vi "5 ch 1 sample minimum resonance scanner (FPGA) fixed pix clock.vi"() -> ()   [LabVIEW 2012]
uses:
  <vilib>/eio/EIONode/EIONode.xnode
  <vilib>/rvi/eio/common/nirviEmuTemplateMethod_errors.vi
  <vilib>/rvi/DataTransferAndStorage/Container/XNode/niFpgaContainer.xnode
  <vilib>/platform/TimedLoop/XDataNode/XDataNode.xnode
  <vilib>/Platform/TimedLoop/XDataNode/nitl_modes.ctl
  <vilib>/Platform/TimedLoop/XDataNode/XDNodeRunTimeDep.lvlib
  <vilib>/Platform/TimedLoop/XDataNode/wakeup.ctl
  <vilib>/Platform/TimedLoop/XDataNode/timing_clust.ctl
  <vilib>/rvi/interface/RandomDataEmulation/nirviRandomDataFpgaReadWriteTemplate.vi
panel:
  in  "lines at once":i16=4999
  in  "samples per half period":i16=4999
  in  "Start Delay (Ticks)":i16 caption="Start delay (Ticks)"
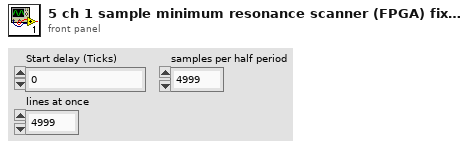
[diagram p1: front panel]
types:
  T1 = typedef "XDNodeRunTimeDep.lvlib/timing_clust.ctl" = cluster{"Expected End [f-1]":u64, "Actual End [f-1]":u64, "Finished Late? [f-1]":bool, "Expected End [i-1]":u64, "Actual End [i-1]":u64, "Finished Late? [i-1]":bool, "Expected Start [i]":u64, "Actual Start [i]":u64, "Expected Start [f]":u64, "Actual Start [f]":u64, "Source Name":string, "Structure Name":string, "Period":i64, "Deadline":i64, "Offset":i64, "Start":i64, "Priority":i32, "Timeout":i32, "Mode":T2, "Wakeup Reason":T3, "Error":errorcluster, "Source Type":string, "Secondary Source Type":string, "Global End Time":u64, "Global Start Time":u64, "Frame Duration":u64, "Iteration Duration":u64, "Assigned CPU":i32, "I/O Scan Engine Mode":u32}
  T2 = typedef "XDNodeRunTimeDep.lvlib/nitl_modes.ctl" = enum32{"No Change", "Process missed periods, maintain original phase", "Discard missed periods, maintain original phase", "Process missed periods, ignore original phase", "Discard missed periods, ignore original phase"}
  T3 = typedef "XDNodeRunTimeDep.lvlib/wakeup.ctl" = enum32{"Normal", "Aborted", "Asynchronous wakeup", "Timing source error", "Timed loop error", "Timeout"}
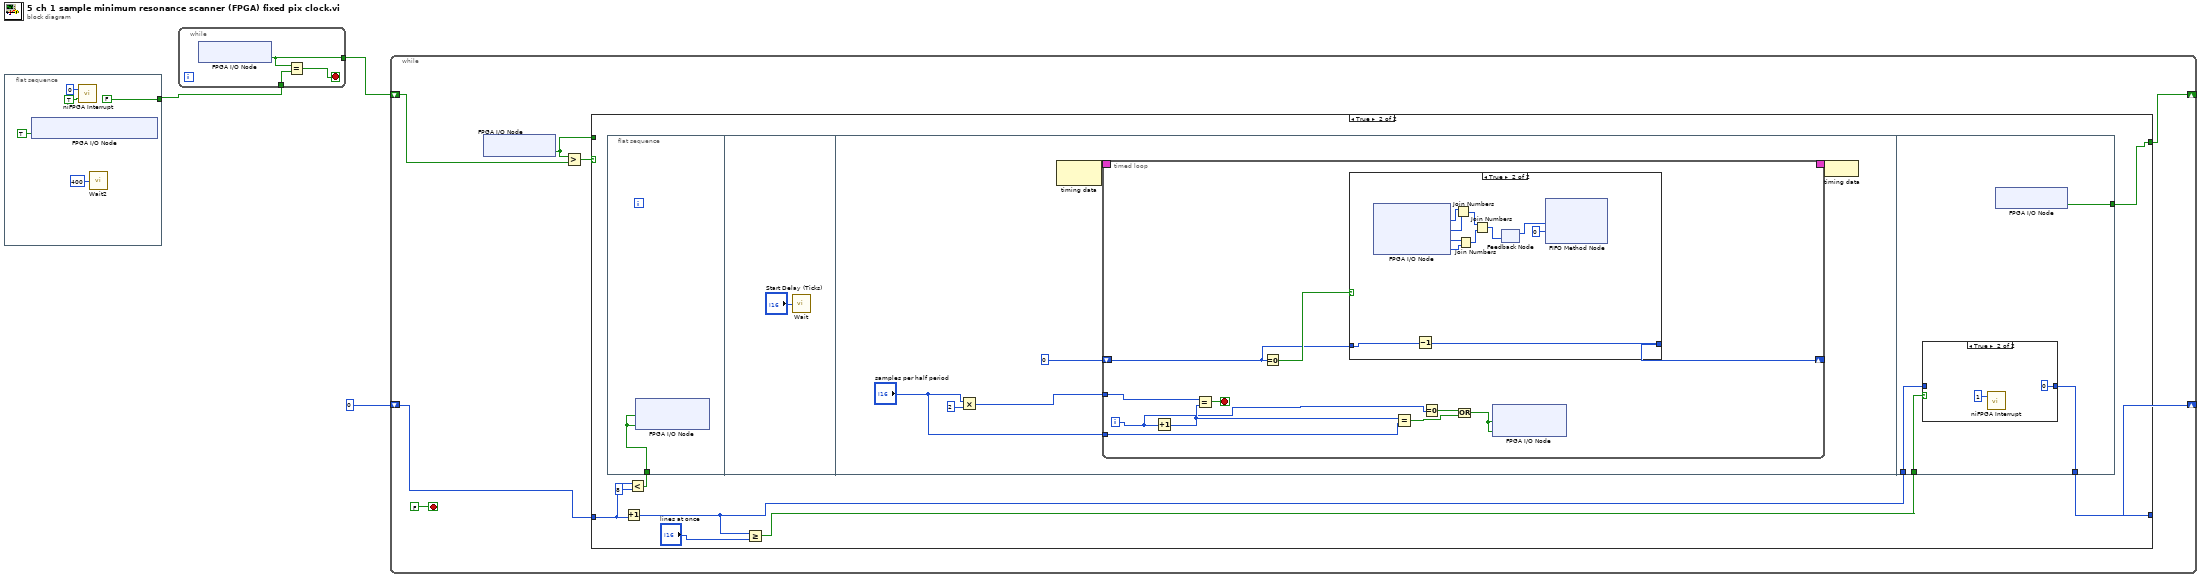
[diagram p0: block diagram]
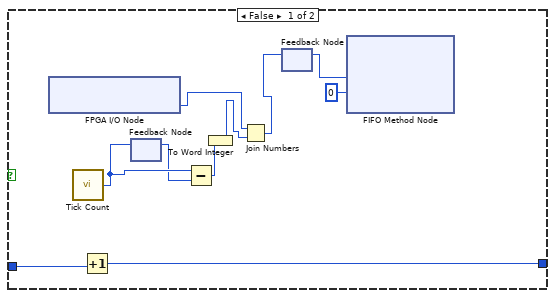
[diagram p3: hidden frame]
diagram:
  n1 = flat-sequence {
    tunnel: [FALSE ("IO Module\\DI 0")] -> w2
    frame #0 {
      n2 = xnode "FPGA I/O Node"("IO Module\\Digital Output Enable"=TRUE ("IO Module\\Digital Output Enable")) -> ()  [unwired: 1 in, 1 out]
      n3 = call <vilib>:"niFPGA Interrupt.vi"("Wait Until Cleared (F)"=TRUE, "IRQ Number (0)"=u8 0) -> ()  [unwired: 1 in]
      n4 = call "Wait2"("Count(mSec)"=u32 400) -> ()  [unwired: 1 out]
    }
  }
  n5 = while {
    tunnel: w2 -> [w11]
    tunnel: [w9] -> w1
    stop <- w10 stop-if-true
    n6 = xnode "FPGA I/O Node"() -> ("IO Module\\DI 0"=w9:bool)  [unwired: 1 in, 1 out]
    n7 = Equal?(x=w9, y=w11) -> (x = y?=w10:bool)
  }
  n8 = while {
    shift-right: [w17] -> _
    shift-left: w1 -> [w18]
    shift-right: [w15] -> _
    shift-left: i16 0 ("IRQ Number (0)") -> [w14]
    stop <- FALSE stop-if-true
    n9 = xnode "FPGA I/O Node"() -> ("IO Module\\DI 0"=w12:bool)  [unwired: 1 in, 1 out]
    n10 = Greater?(x=w12, y=w18) -> (0:w13:bool)
    n11 = case shown="True" w13 {
      tunnel: [w19 w21] -> w17
      tunnel: w14 -> [w20 w24]
      tunnel: [w20 w26] -> w15
      tunnel: w12 -> [w19 _]
      frame False {
      }
      frame True {
        n12 = flat-sequence {
          tunnel: w22 -> [w29]
          tunnel: w28 -> [w76]
          tunnel: w27 -> [w75]
          tunnel: [w74] -> w26
          tunnel: [w73] -> w21
          frame #0 {
            n13 = xnode "FPGA I/O Node"("PXI_Trig2"=w29, "IO Module\\D0 2"=w29) -> ()  [unwired: 2 in, 2 out]
          }
          frame #1 {
            n14 = call "Wait"("Count(Ticks)"="Start Delay (Ticks)") -> ()  [unwired: 1 out]
          }
          frame #2 {
            n15 = Multiply(x="samples per half period", y=i16 2) -> (x*y=w35:i16)
            n16 = node-c288() -> (w34:T1)  [unwired: 1 in]
            n17 = timed-loop {
              tunnel: w35 -> [w46]
              timing: w34 -> [_]
              timing-out: [_] -> w33
              shift-right: [w43] -> _
              shift-left: 0 ("Timeout") -> [w44]
              tunnel: "samples per half period" -> [w38]
              i -> [w37]
              stop <- w47 stop-if-true
              n18 = Increment(x=w37) -> (x+1=w39:i32)
              n19 = Equal?(x=w46, y=w39) -> (x = y?=w47:bool)
              n20 = Equal To 0?(x=w44) -> (x = 0?=w45:bool)
              n21 = case shown="True" w45 {
                tunnel: w44 -> [w57 w67]
                tunnel: [w56 w66] -> w43
                frame False {
                  n22 = xnode "FPGA I/O Node"() -> ("IO Module\\AI B8"=w50:i16)  [unwired: 1 in, 1 out]
                  n23 = call "Tick Count"() -> ("Tick Count(Ticks)"=w54:u32)
                  n24 = Increment(x=w57) -> (x+1=w56:i32)
                  n25 = feedback #1() -> (w53:u32)  [unwired: 1 in]
                  n26 = feedback-in #1(w54) -> ()
                  n27 = Subtract(x=w54, y=w53) -> (x-y=w52:u32)
                  n28 = To Word Integer(number=w52) -> (16bit integer=w49:i16)
                  n29 = Join Numbers(hi=w50, lo=w49) -> ((hi.lo)=w48:u32)
                  n30 = feedback-in #2(w48) -> ()
                  n31 = feedback #2() -> (w55:u32)  [unwired: 1 in]
                  n32 = xnode ("FIFO Method Node")("Element"=w55, "Timeout"=0) -> ()  [unwired: 1 in, 2 out]
                }
                frame True {
                  n33 = xnode "FPGA I/O Node"() -> ("IO Module\\AI A0"=w64:i16, "IO Module\\AI A1"=w63:i16, "IO Module\\AI A3"=w62:i16, "IO Module\\AI A6"=w61:i16)  [unwired: 4 in, 4 out]
                  n34 = Decrement(x=w67) -> (x-1=w66:i32)
                  n35 = Join Numbers(hi=w64, lo=w63) -> ((hi.lo)=w59:u32)
                  n36 = Join Numbers(hi=w62, lo=w61) -> ((hi.lo)=w60:u32)
                  n37 = Join Numbers(hi=w59, lo=w60) -> ((hi.lo)=w58:u64)
                  n38 = feedback-in #3(w58) -> ()
                  n39 = feedback #3() -> (w65:u64)  [unwired: 1 in]
                  n40 = xnode ("FIFO Method Node")("Element"=w65, "Timeout"=0) -> ()  [unwired: 1 in, 2 out]
                }
              }
              n41 = Equal?(x=w39, y=w38) -> (x = y?=w41:bool)
              n42 = Equal To 0?(x=w37) -> (x = 0?=w42:bool)
              n43 = Or(x=w42, y=w41) -> (x .or. y?=w40:bool)
              n44 = xnode "FPGA I/O Node"("IO Module\\D0 1"=w40, "PXI_Trig1"=w40) -> ()  [unwired: 2 in, 2 out]
            }
            n45 = node-c288(w33) -> ()
          }
          frame #3 {
            n46 = case shown="True" w75 {
              tunnel: w76 -> [w77 _]
              tunnel: [w77 u8 0] -> w74
              frame False {
              }
              frame True {
                n47 = call <vilib>:"niFPGA Interrupt.vi"("IRQ Number (0)"=u8 1) -> ()  [unwired: 2 in]
              }
            }
            n48 = xnode "FPGA I/O Node"() -> ("IO Module\\DI 0"=w73:bool)  [unwired: 1 in, 1 out]
          }
        }
        n49 = Increment(x=w24) -> (x+1=w28:i16)
        n50 = Less?(x=w24, y=i16 8) -> (x < y?=w22:bool)
        n51 = Greater Or Equal?(x=w28, y="lines at once") -> (x >= y?=w27:bool)
      }
    }
  }
